vi "Get Build Specification Version (path).vi"(8 "error in (no error)":errorcluster, 9 "Name of target (My Computer)":string="My Computer", 10 "Name of build specification":string, 11 "Path to project":path) -> (0 "error out":errorcluster, 4 "Build Specification Version":T1)   [LabVIEW 2020, in "NI_App_Builder_API.lvlib"]
doc: "Gets the version information of a build specification. This VI returns the <B>Major, Minor, Fix</B>, and <B>Build</B> version numbers, which correspond to the version numbers on the <B>Version Information</B> page of the properties dialog box for the build specification."
uses:
  <vilib>/AppBuilder/AB_API_Simple/NI_App_Builder_API.lvlib
  <vilib>/AppBuilder/AB_API_Simple/Build Specification Version.ctl
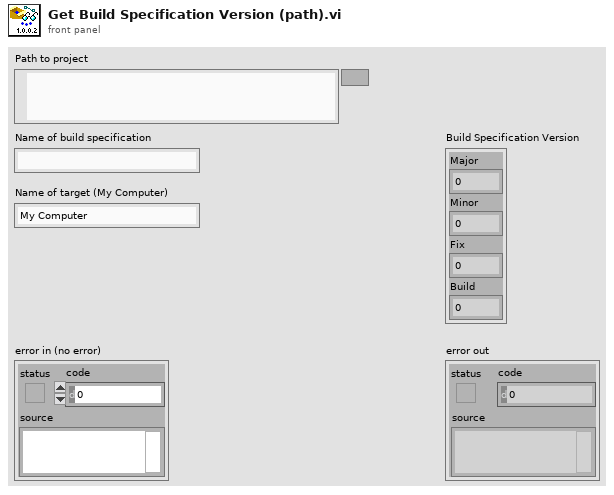
[diagram p1: front panel]
types:
  T1 = typedef "NI_App_Builder_API.lvlib/Build Specification Version.ctl" = cluster{"Major":u16, "Minor":u16, "Fix":u16, "Build":u16}
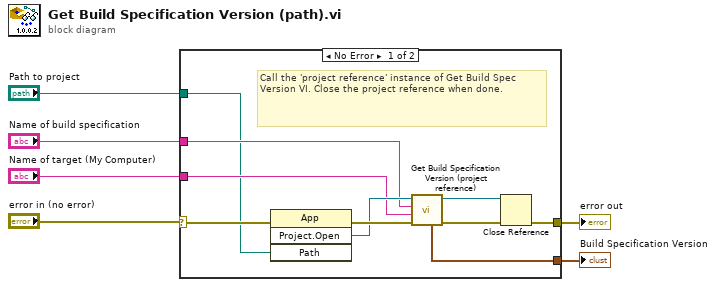
[diagram p0: block diagram]
diagram:
  n1 = case shown="No Error" "error in (no error)" {
    selector: "error in (no error)" -> [w16 w17]
    tunnel: "Path to project" -> [w8 _]
    tunnel: "Name of target (My Computer)" -> [w9 _]
    tunnel: "Name of build specification" -> [w10 _]
    tunnel: [w7 _] -> w4
    tunnel: [w11 w17] -> w3
    frame No Error {
      # "Call the 'project reference' instance of Get Build Spec Version VI. Close the project reference when done."
      n2 = invoke class="App" method="Project.Open"(error in=w16, "Path"=w8) -> (error out=w15:errorcluster, "Project:Open"=w14:refnum<vi>)  [unwired: 2 in, 2 out]
      n3 = call <vilib>:"Get Build Specification Version (project reference).vi"("error in (no error)"=w15, "Name of target (My Computer)"=w9, "Name of build specification"=w10, "Project reference"=w14) -> ("error out"=w13:errorcluster, "dup Project reference"=w12:refnum<vi>, "Build Specification Version"=w7:T1)  [unwired: 5 in]
      n4 = Close Reference(reference=w12, error in (no error)=w13) -> (error out=w11:errorcluster)
    }
    frame Error {
    }
  }
  "error out" <- w3
  "Build Specification Version" <- w4
